vi "AUTO SIMPLE.vi"(8 "error in (no error)":errorcluster, 10 "auto command list":T1={"SHOOT\nFIRST"=FALSE, "wait to\nSHOOT (ms)"=1500, "run\nINTAKE"=FALSE, "DRIVE BRNG (deg)"=0.0, "DRIVE OUT\nVBus"=0.65, "TIME to\nDRIVE OUT (ms)"=1750, "pause after\ndrive out (ms)"=500, "SHOOT\nAGAIN"=FALSE, "DRIVE IN\nVBus"=0.0, "TIME to\nDRIVE IN (ms)"=0} {"DRIVE IN\nVBus" format="%#_13g"; "DRIVE OUT\nVBus" format="%#_13g"}) -> (0 "error out":errorcluster)   [LabVIEW 2023]
uses:
  ctrl defs/ctrl AUTO SIMPLE STEP.ctl
  ctrl defs/ctrl AUTO STEPS.ctl
  ctrl defs/ctrl FRONT FACE selector.ctl
  Global odometry.vi
  Global stack names.vi
  <vilib>/Rock Robotics/Network Tables/NT Write Boolean.vi
  <vilib>/Utility/semaphor.llb/Obtain Semaphore Reference.vi
  <vilib>/Rock Robotics/WPI/ThirdParty/JAS_Junk/TrajLib/Timer_Reset.vi
  <vilib>/Rock Robotics/WPI/ThirdParty/JAS_Junk/TrajLib/Trajectory_Library.lvlib
panel:
  out "pause after\ndrive out (ms)":u32
  out "TIME to\nDRIVE IN (ms)":u32
  out "DRIVE IN\nVBus":dbl
  out "DRIVE BRNG (deg)":u32
  out "wait to\nSHOOT (ms)":u32
  out "SHOOT\nAGAIN":bool
  out "TIME to\nDRIVE OUT (ms)":u32
  out "DRIVE OUT\nVBus":dbl
  out "run\nINTAKE":bool
  out "SHOOT\nFIRST":bool
  in  "EXIT LOOP":bool
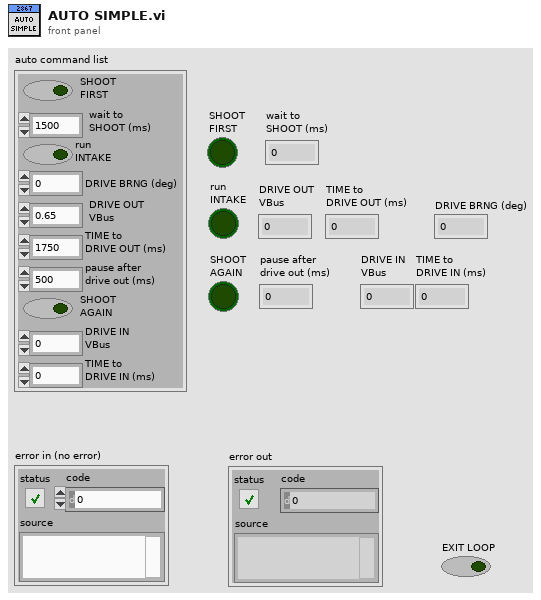
[diagram p1: front panel]
types:
  T1 = typedef "ctrl AUTO SIMPLE STEP.ctl" = cluster{"SHOOT\nFIRST":bool, "wait to\nSHOOT (ms)":u32, "run\nINTAKE":bool, "DRIVE BRNG (deg)":dbl, "DRIVE OUT\nVBus":dbl, "TIME to\nDRIVE OUT (ms)":u32, "pause after\ndrive out (ms)":u32, "SHOOT\nAGAIN":bool, "DRIVE IN\nVBus":dbl, "TIME to\nDRIVE IN (ms)":u32}
  T2 = typedef "ctrl FRONT FACE selector.ctl" = enum16{"intake side", "shooter side"}
  T3 = typedef "ctrl AUTO STEPS.ctl" = enum16{"SHOOT", "INTAKE", "ROLL OUT", "DRIVE UP", "SHOOT AGAIN", "END", "PAUSE to SHOOT", "END DRIVE"}
  T4 = typedef "ctrl stack - INTAKE SHOOTER.ctl" = cluster{"INTAKE STATE":string, "RUN INTAKE?":string, "RUN REVERSE?":string, "NOTE LOADED?":string, "SHOOTER STATE":string, "SHOOTER FIRE?":string, "SHOOT AMP?":string, "EXTEND FLAP?":string, "LOOKING for NOTE":string, "OVERIDE NOTE CHECK":string}
  T5 = typedef "Trajectory_Library.lvlib/TIMER.ctl" = cluster{"StartTime":dbl, "Accumulated TIme":dbl, "Running":bool, "semaphore":T6}
  T6 = typedef "Semaphore RefNum" = refnum<k1>
  T7 = typedef "ctrl driver input.ctl" = cluster{"Jx":dbl, "Jy":dbl, "Jr ":dbl, "R":dbl, "theta (deg)":dbl, "theta (rad)":dbl, "PARK":bool}
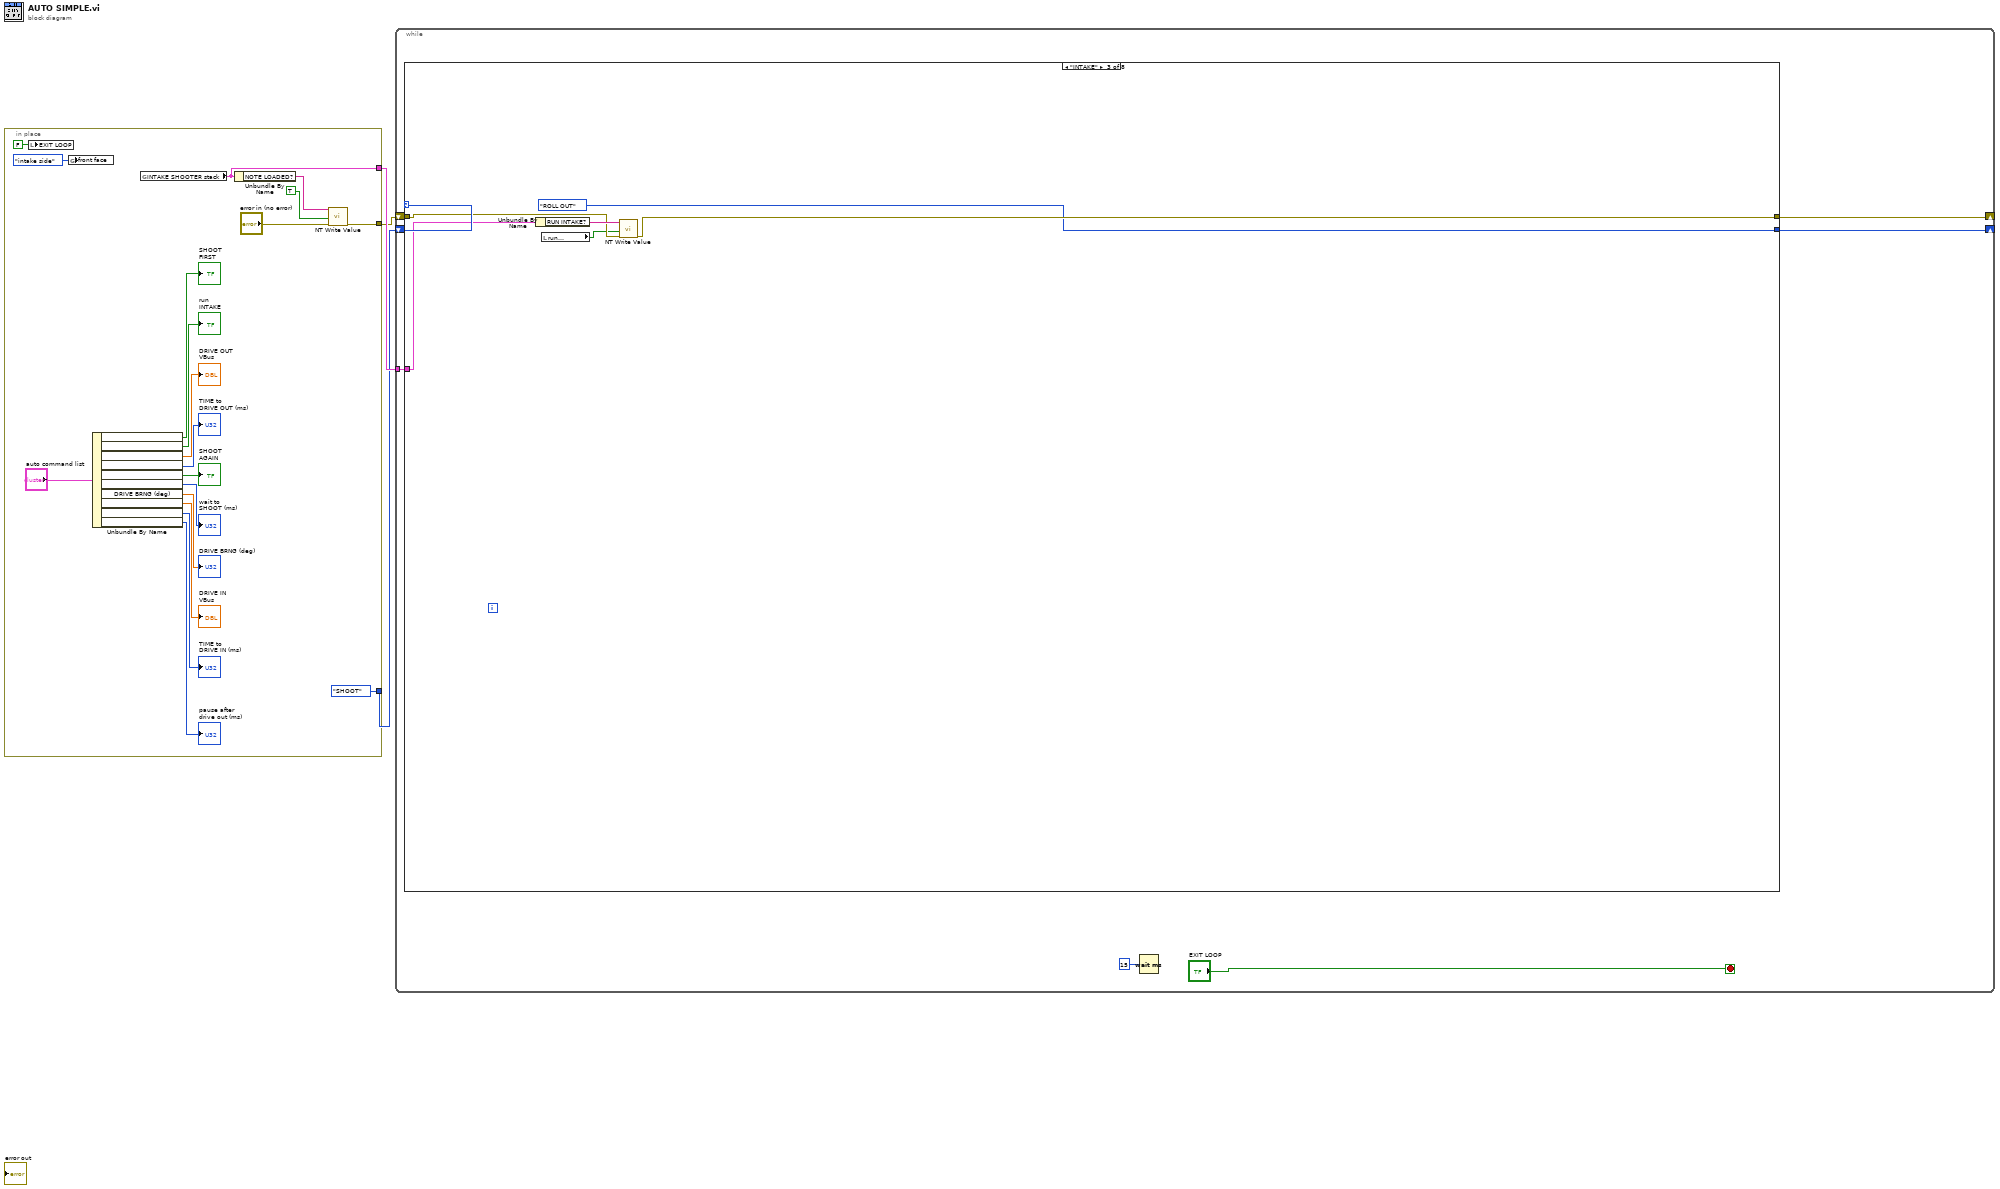
[diagram p0: block diagram]
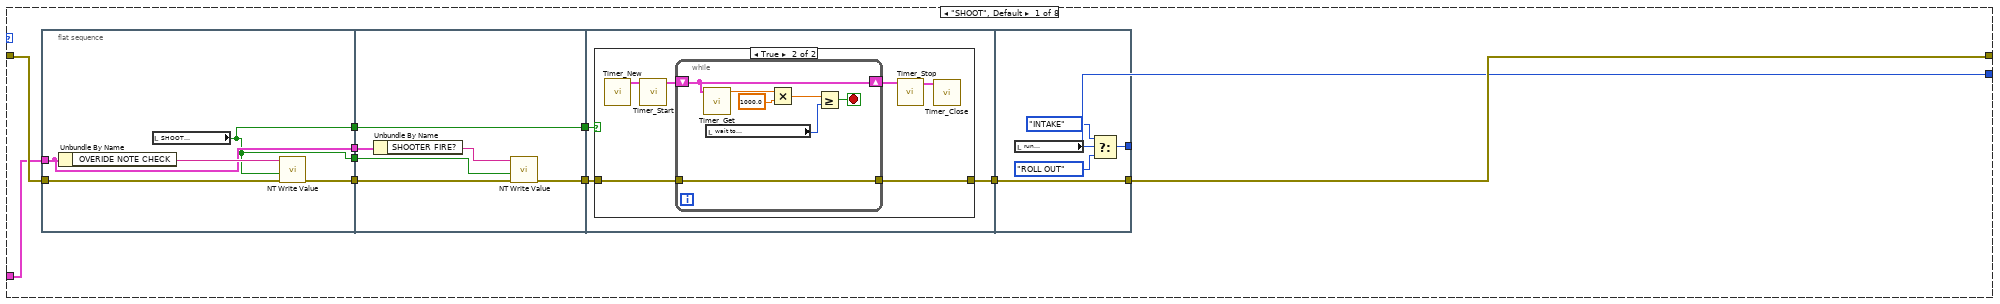
[diagram p2: hidden frame]
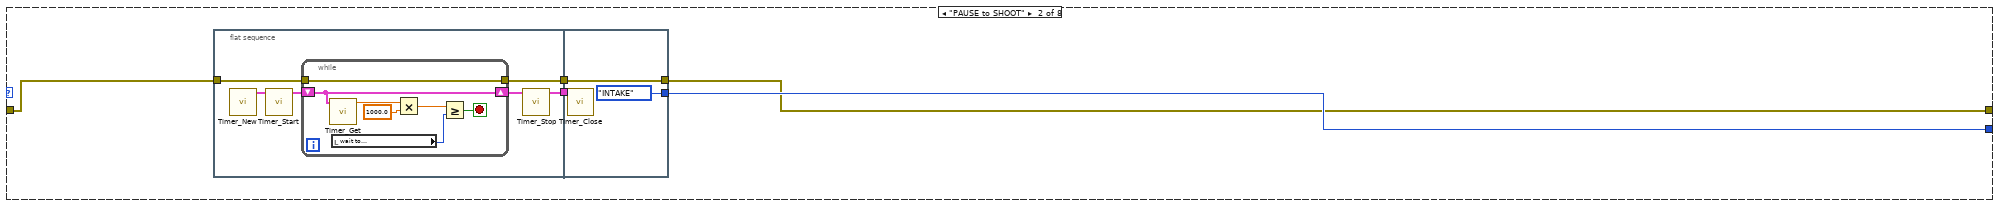
[diagram p4: hidden frame]
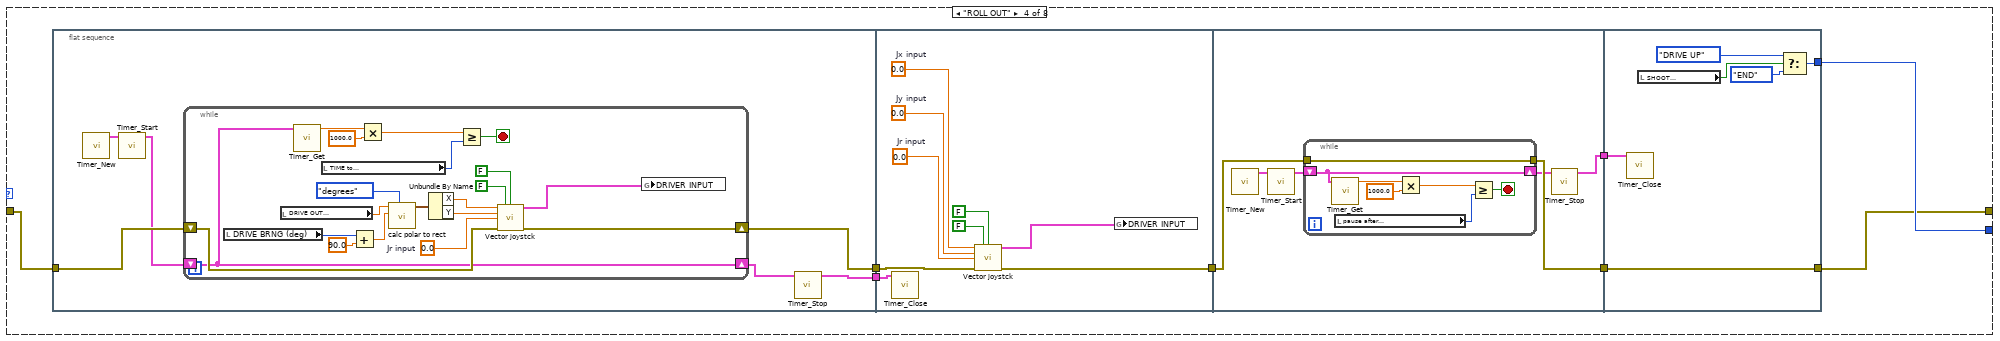
[diagram p5: hidden frame]
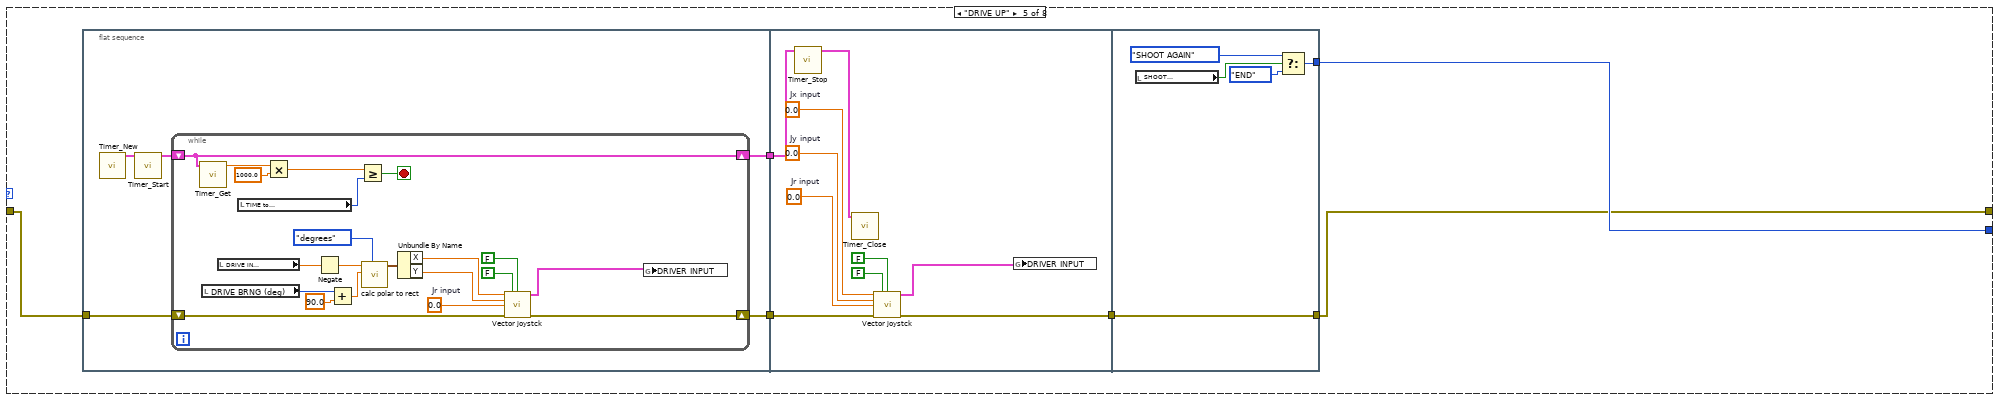
[diagram p6: hidden frame]
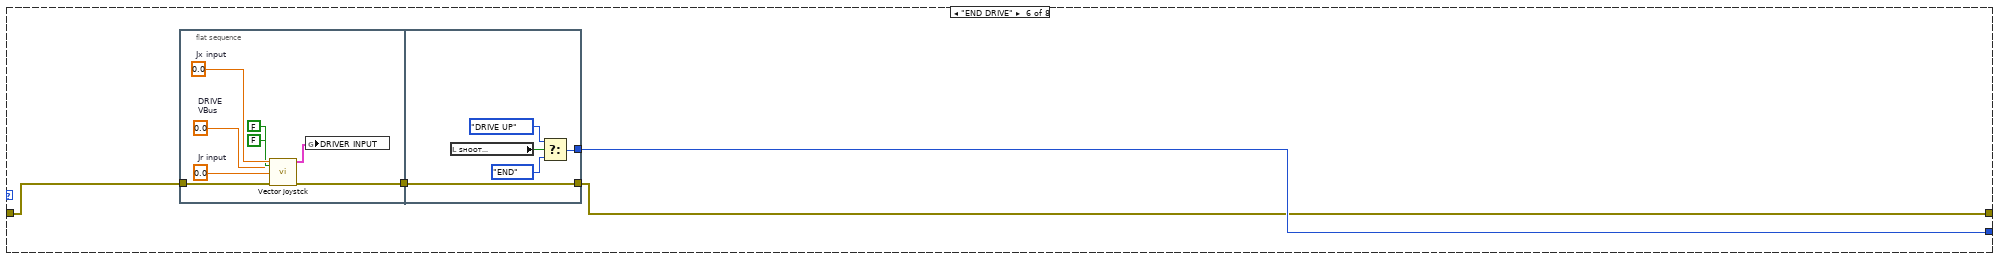
[diagram p7: hidden frame]
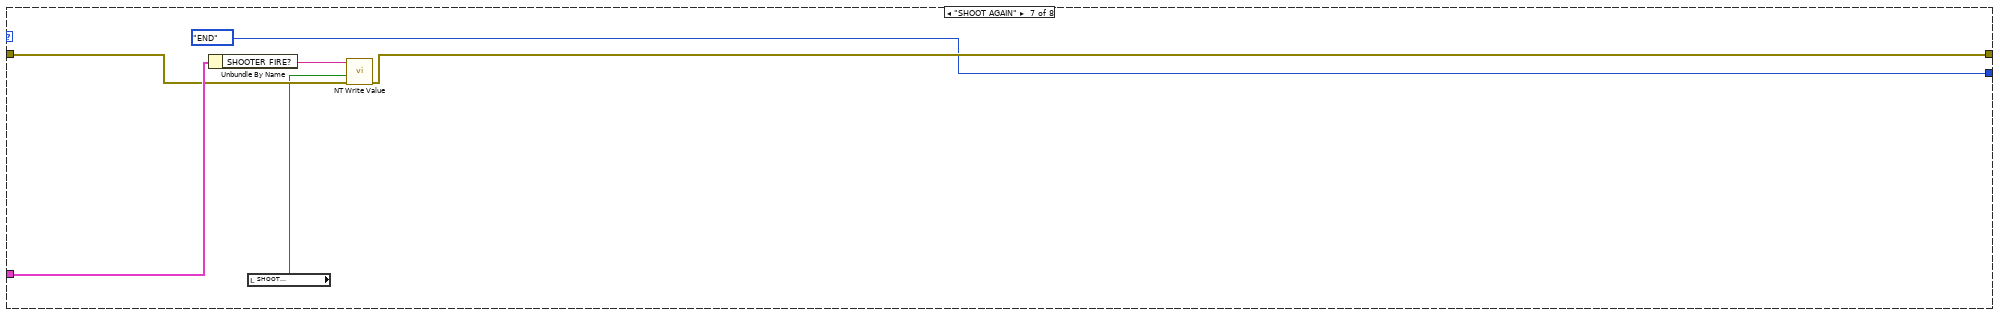
[diagram p8: hidden frame]
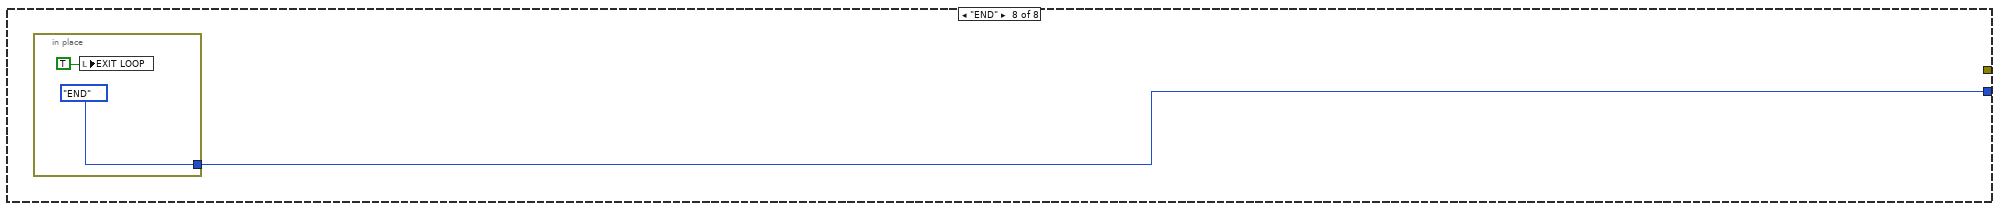
[diagram p9: hidden frame]
diagram:
  n1 = in-place {
    in-place-border: [w14] -> w3
    in-place-border: [w9] -> w2
    in-place-border: [ctrl_AUTO_STEPS."SHOOT"] -> w1
    n2 = local write "EXIT LOOP"(FALSE ("EXIT LOOP")) -> ()
    n3 = global write "Global odometry.vi" "front face"(ctrl_FRONT_FACE_selector."intake side" ("front face")) -> ()
    n4 = Unbundle By Name("auto command list") -> ("SHOOT\nFIRST"=→"SHOOT\nFIRST":bool, "run\nINTAKE"=→"run\nINTAKE":bool, "DRIVE OUT\nVBus"=→"DRIVE OUT\nVBus":dbl, "TIME to\nDRIVE OUT (ms)"=→"TIME to\nDRIVE OUT (ms)":u32, "SHOOT\nAGAIN"=→"SHOOT\nAGAIN":bool, "wait to\nSHOOT (ms)"=→"wait to\nSHOOT (ms)":u32, "DRIVE BRNG (deg)"=→"DRIVE BRNG (deg)":dbl, "DRIVE IN\nVBus"=→"DRIVE IN\nVBus":dbl, "TIME to\nDRIVE IN (ms)"=→"TIME to\nDRIVE IN (ms)":u32, "pause after\ndrive out (ms)"=→"pause after\ndrive out (ms)":u32)
    n5 = global read "Global stack names.vi" "INTAKE SHOOTER stack"() -> (w14:T4)
    n6 = Unbundle By Name(w14) -> ("NOTE LOADED?"=w13:string)
    n7 = call-poly <vilib>:"NT Write Value.vi"("error in"="error in (no error)", "value"=TRUE, "name"=w13) -> ("error out"=w9:errorcluster)  [unwired: 8 in]
  }
  n8 = while {
    shift-right: [w27] -> _
    shift-left: w2 -> [w29]
    tunnel: w3 -> [w28]
    shift-right: [w25] -> _
    shift-left: w1 -> [w26]
    stop <- "EXIT LOOP" stop-if-true
    n9 = case shown="\"INTAKE\"" w26 {
      tunnel: w28 -> [w37 _ w98 _ _ _ w231 _]
      tunnel: [w40 w74 w96 w105 w165 w210 w229 _] -> w27
      tunnel: w29 -> [w39 w76 w97 w106 w166 w211 w228 _]
      tunnel: [w38 w77 ctrl_AUTO_STEPS."ROLL OUT" w107 w167 w212 ctrl_AUTO_STEPS."END" w232] -> w25
      frame "SHOOT", Default {
        n10 = flat-sequence {
          tunnel: w39 -> [w45]
          tunnel: w37 -> [w42]
          tunnel: [w43] -> w36
          tunnel: [w41] -> w35
          tunnel: [w42] -> w34
          tunnel: [w41] -> w31
          tunnel: w36 -> [w50]
          tunnel: w35 -> [w49]
          tunnel: w34 -> [w47]
          tunnel: [w48] -> w33
          tunnel: w31 -> [w46]
          tunnel: [w46] -> w30
          tunnel: w33 -> [w54]
          tunnel: [w53] -> w32
          tunnel: w30 -> [w52]
          tunnel: [w69] -> w38
          tunnel: [w72] -> w40
          tunnel: w32 -> [w72]
          frame #0 {
            n11 = Unbundle By Name(w42) -> ("OVERIDE NOTE CHECK"=w44:string)
            n12 = local read "SHOOT\nFIRST"() -> (w41:bool)
            n13 = call-poly <vilib>:"NT Write Value.vi"("error in"=w45, "value"=w41, "name"=w44) -> ("error out"=w43:errorcluster)  [unwired: 8 in]
          }
          frame #1 {
            n14 = Unbundle By Name(w47) -> ("SHOOTER FIRE?"=w51:string)
            n15 = call-poly <vilib>:"NT Write Value.vi"("error in"=w50, "value"=w49, "name"=w51) -> ("error out"=w48:errorcluster)  [unwired: 8 in]
          }
          frame #2 {
            n16 = case shown="True" w52 {
              tunnel: w54 -> [_ w57]
              tunnel: [_ w56] -> w53
              frame False {
              }
              frame True {
                n17 = call <vilib>:"Timer_New.vi"() -> ("TIMER"=w58:T5)  [unwired: 11 in]
                n18 = call <vilib>:"Timer_Start.vi"("in Timer"=w58) -> ("out Timer"=w59:T5)  [unwired: 10 in]
                n19 = while {
                  shift-right: [w67] -> w60
                  shift-left: w59 -> [w67]
                  tunnel: w57 -> [w61]
                  tunnel: [w61] -> w56
                  stop <- w66 stop-if-true
                  n20 = call <vilib>:"Timer_Get.vi"("TIMER"=w67) -> ("CurrentTImer"=w65:dbl)  [unwired: 10 in]
                  n21 = local read "wait to\nSHOOT (ms)"() -> (w64:u32)
                  n22 = Multiply(x=w65, y=1000.0) -> (x*y=w63:dbl)
                  n23 = Greater Or Equal?(x=w63, y=w64) -> (x >= y?=w66:bool)
                }
                n24 = call <vilib>:"Timer_Stop.vi"("in Timer"=w60) -> ("out Timer"=w55:T5)  [unwired: 10 in]
                n25 = call <vilib>:"Timer_Close.vi"("TIMER"=w55) -> ()  [unwired: 11 in]
              }
            }
          }
          frame #3 {
            n26 = local read "run\nINTAKE"() -> (w68:bool)
            n27 = Select(t=ctrl_AUTO_STEPS."INTAKE", s=w68, f=ctrl_AUTO_STEPS."ROLL OUT") -> (s? t:f=w69:T3)
          }
        }
      }
      frame "PAUSE to SHOOT" {
        n28 = flat-sequence {
          tunnel: w76 -> [w80]
          tunnel: [w79] -> w75
          tunnel: [w78] -> w73
          tunnel: [ctrl_AUTO_STEPS."INTAKE"] -> w77
          tunnel: w75 -> [w92]
          tunnel: [w92] -> w74
          tunnel: w73 -> [w91]
          frame #0 {
            n29 = call <vilib>:"Timer_New.vi"() -> ("TIMER"=w81:T5)  [unwired: 11 in]
            n30 = call <vilib>:"Timer_Start.vi"("in Timer"=w81) -> ("out Timer"=w82:T5)  [unwired: 10 in]
            n31 = while {
              shift-right: [w86] -> w83
              shift-left: w82 -> [w86]
              tunnel: w80 -> [w84]
              tunnel: [w84] -> w79
              stop <- w85 stop-if-true
              n32 = call <vilib>:"Timer_Get.vi"("TIMER"=w86) -> ("CurrentTImer"=w90:dbl)  [unwired: 10 in]
              n33 = local read "wait to\nSHOOT (ms)"() -> (w89:u32)
              n34 = Multiply(x=w90, y=1000.0) -> (x*y=w88:dbl)
              n35 = Greater Or Equal?(x=w88, y=w89) -> (x >= y?=w85:bool)
            }
            n36 = call <vilib>:"Timer_Stop.vi"("in Timer"=w83) -> ("out Timer"=w78:T5)  [unwired: 10 in]
          }
          frame #1 {
            n37 = call <vilib>:"Timer_Close.vi"("TIMER"=w91) -> ()  [unwired: 11 in]
          }
        }
      }
      frame "INTAKE" {
        n38 = Unbundle By Name(w98) -> ("RUN INTAKE?"=w99:string)
        n39 = local read "run\nINTAKE"() -> (w94:bool)
        n40 = call-poly <vilib>:"NT Write Value.vi"("error in"=w97, "value"=w94, "name"=w99) -> ("error out"=w96:errorcluster)  [unwired: 8 in]
      }
      frame "ROLL OUT" {
        n41 = flat-sequence {
          tunnel: w106 -> [w113]
          tunnel: [w112] -> w102
          tunnel: [w108] -> w101
          tunnel: w102 -> [w137]
          tunnel: [w136] -> w104
          tunnel: w101 -> [w135]
          tunnel: w104 -> [w147]
          tunnel: [w146] -> w103
          tunnel: [w143] -> w100
          tunnel: [w161] -> w107
          tunnel: w103 -> [w158]
          tunnel: [w158] -> w105
          tunnel: w100 -> [w156]
          frame #0 {
            n42 = call <vilib>:"Timer_New.vi"() -> ("TIMER"=w111:T5)  [unwired: 11 in]
            n43 = call <vilib>:"Timer_Start.vi"("in Timer"=w111) -> ("out Timer"=w110:T5)  [unwired: 10 in]
            n44 = while {
              shift-right: [w130] -> w112
              shift-left: w113 -> [w131]
              shift-right: [w117] -> w109
              shift-left: w110 -> [w117]
              stop <- w115 stop-if-true
              w129 = 0.0  # Jr input
              n45 = local read "DRIVE BRNG (deg)"() -> (w125:u32)
              n46 = local read "DRIVE OUT\nVBus"() -> (w127:dbl)
              n47 = call <vilib>:"Timer_Get.vi"("TIMER"=w117) -> ("CurrentTImer"=w119:dbl)  [unwired: 10 in]
              n48 = local read "TIME to\nDRIVE OUT (ms)"() -> (w116:u32)
              n49 = Add(x=w125, y=90.0) -> (x+y=w126:dbl)
              n50 = Multiply(x=w119, y=1000.0) -> (x*y=w120:dbl)
              n51 = call "calc polar to rect.vi"("units"=enum16{"degrees", "radians"}."degrees", "angle"=w126, "mag"=w127) -> ("XY"=w128:cluster{"X":dbl, "Y":dbl})  [unwired: 8 in]
              n52 = Unbundle By Name(w128) -> ("X"=w122:dbl, "Y"=w121:dbl)
              n53 = Greater Or Equal?(x=w120, y=w116) -> (x >= y?=w115:bool)
              n54 = call "Vector joystck.vi"("Jx input"=w122, "apply\nFILTER"=FALSE ("apply\nFILTER"), "Reset\nFILTER"=FALSE ("Reset\nFILTER"), "Jy input"=w121, "Jr input"=w129, "error in (no error)"=w131) -> ("output cluster"=w114:T7, "error out"=w130:errorcluster)  [unwired: 8 in]
              n55 = global write "Global odometry.vi" "DRIVER INPUT"(w114) -> ()
            }
            n56 = call <vilib>:"Timer_Stop.vi"("in Timer"=w109) -> ("out Timer"=w108:T5)  [unwired: 10 in]
          }
          frame #1 {
            w138 = 0.0  # Jy input
            w139 = 0.0  # Jr input
            w142 = 0.0  # Jx input
            n57 = call <vilib>:"Timer_Close.vi"("TIMER"=w135) -> ()  [unwired: 11 in]
            n58 = call "Vector joystck.vi"("Jx input"=w142, "apply\nFILTER"=FALSE ("apply\nFILTER"), "Reset\nFILTER"=FALSE ("Reset\nFILTER"), "Jy input"=w138, "Jr input"=w139, "error in (no error)"=w137) -> ("output cluster"=w134:T7, "error out"=w136:errorcluster)  [unwired: 8 in]
            n59 = global write "Global odometry.vi" "DRIVER INPUT"(w134) -> ()
          }
          frame #2 {
            n60 = call <vilib>:"Timer_New.vi"() -> ("TIMER"=w148:T5)  [unwired: 11 in]
            n61 = call <vilib>:"Timer_Start.vi"("in Timer"=w148) -> ("out Timer"=w145:T5)  [unwired: 10 in]
            n62 = while {
              tunnel: w147 -> [w153]
              tunnel: [w153] -> w146
              shift-right: [w152] -> w144
              shift-left: w145 -> [w152]
              stop <- w155 stop-if-true
              n63 = call <vilib>:"Timer_Get.vi"("TIMER"=w152) -> ("CurrentTImer"=w151:dbl)  [unwired: 10 in]
              n64 = local read "pause after\ndrive out (ms)"() -> (w154:u32)
              n65 = Multiply(x=w151, y=1000.0) -> (x*y=w150:dbl)
              n66 = Greater Or Equal?(x=w150, y=w154) -> (x >= y?=w155:bool)
            }
            n67 = call <vilib>:"Timer_Stop.vi"("in Timer"=w144) -> ("out Timer"=w143:T5)  [unwired: 10 in]
          }
          frame #3 {
            n68 = call <vilib>:"Timer_Close.vi"("TIMER"=w156) -> ()  [unwired: 11 in]
            n69 = local read "SHOOT\nAGAIN"() -> (w157:bool)
            n70 = Select(t=ctrl_AUTO_STEPS."DRIVE UP", s=w157, f=ctrl_AUTO_STEPS."END") -> (s? t:f=w161:T3)
          }
        }
      }
      frame "DRIVE UP" {
        n71 = flat-sequence {
          tunnel: w166 -> [w172]
          tunnel: [w171] -> w163
          tunnel: [w168] -> w162
          tunnel: w163 -> [w198]
          tunnel: [w197] -> w164
          tunnel: w162 -> [w195]
          tunnel: [w208] -> w167
          tunnel: w164 -> [w205]
          tunnel: [w205] -> w165
          frame #0 {
            n72 = call <vilib>:"Timer_New.vi"() -> ("TIMER"=w170:T5)  [unwired: 11 in]
            n73 = call <vilib>:"Timer_Start.vi"("in Timer"=w170) -> ("out Timer"=w169:T5)  [unwired: 10 in]
            n74 = while {
              shift-right: [w189] -> w171
              shift-left: w172 -> [w190]
              shift-right: [w179] -> w168
              shift-left: w169 -> [w179]
              stop <- w178 stop-if-true
              w191 = 0.0  # Jr input
              n75 = call <vilib>:"Timer_Get.vi"("TIMER"=w179) -> ("CurrentTImer"=w177:dbl)  [unwired: 10 in]
              n76 = local read "DRIVE BRNG (deg)"() -> (w188:u32)
              n77 = local read "DRIVE IN\nVBus"() -> (w186:dbl)
              n78 = local read "TIME to\nDRIVE IN (ms)"() -> (w174:u32)
              n79 = Multiply(x=w177, y=1000.0) -> (x*y=w176:dbl)
              n80 = Negate(x=w186) -> (-x=w187:dbl)
              n81 = Add(x=w188, y=90.0) -> (x+y=w185:dbl)
              n82 = Greater Or Equal?(x=w176, y=w174) -> (x >= y?=w178:bool)
              n83 = call "calc polar to rect.vi"("units"=enum16{"degrees", "radians"}."degrees", "angle"=w185, "mag"=w187) -> ("XY"=w184:cluster{"X":dbl, "Y":dbl})  [unwired: 8 in]
              n84 = Unbundle By Name(w184) -> ("X"=w181:dbl, "Y"=w180:dbl)
              n85 = call "Vector joystck.vi"("Jx input"=w181, "apply\nFILTER"=FALSE ("apply\nFILTER"), "Reset\nFILTER"=FALSE ("Reset\nFILTER"), "Jy input"=w180, "Jr input"=w191, "error in (no error)"=w190) -> ("output cluster"=w173:T7, "error out"=w189:errorcluster)  [unwired: 8 in]
              n86 = global write "Global odometry.vi" "DRIVER INPUT"(w173) -> ()
            }
          }
          frame #1 {
            w199 = 0.0  # Jy input
            w200 = 0.0  # Jr input
            w203 = 0.0  # Jx input
            n87 = call <vilib>:"Timer_Stop.vi"("in Timer"=w195) -> ("out Timer"=w196:T5)  [unwired: 10 in]
            n88 = call <vilib>:"Timer_Close.vi"("TIMER"=w196) -> ()  [unwired: 11 in]
            n89 = call "Vector joystck.vi"("Jx input"=w203, "apply\nFILTER"=FALSE ("apply\nFILTER"), "Reset\nFILTER"=FALSE ("Reset\nFILTER"), "Jy input"=w199, "Jr input"=w200, "error in (no error)"=w198) -> ("output cluster"=w194:T7, "error out"=w197:errorcluster)  [unwired: 8 in]
            n90 = global write "Global odometry.vi" "DRIVER INPUT"(w194) -> ()
          }
          frame #2 {
            n91 = local read "SHOOT\nAGAIN"() -> (w204:bool)
            n92 = Select(t=ctrl_AUTO_STEPS."SHOOT AGAIN", s=w204, f=ctrl_AUTO_STEPS."END") -> (s? t:f=w208:T3)
          }
        }
      }
      frame "END DRIVE" {
        n93 = flat-sequence {
          tunnel: w211 -> [w215]
          tunnel: [w214] -> w209
          tunnel: [w225] -> w212
          tunnel: w209 -> [w222]
          tunnel: [w222] -> w210
          frame #0 {
            w217 = 0.0  # DRIVE VBus
            w216 = 0.0  # Jr input
            w220 = 0.0  # Jx input
            n94 = call "Vector joystck.vi"("Jx input"=w220, "apply\nFILTER"=FALSE ("apply\nFILTER"), "Reset\nFILTER"=FALSE ("Reset\nFILTER"), "Jy input"=w217, "Jr input"=w216, "error in (no error)"=w215) -> ("output cluster"=w213:T7, "error out"=w214:errorcluster)  [unwired: 8 in]
            n95 = global write "Global odometry.vi" "DRIVER INPUT"(w213) -> ()
          }
          frame #1 {
            n96 = local read "SHOOT\nAGAIN"() -> (w221:bool)
            n97 = Select(t=ctrl_AUTO_STEPS."DRIVE UP", s=w221, f=ctrl_AUTO_STEPS."END") -> (s? t:f=w225:T3)
          }
        }
      }
      frame "SHOOT AGAIN" {
        n98 = Unbundle By Name(w231) -> ("SHOOTER FIRE?"=w230:string)
        n99 = local read "SHOOT\nAGAIN"() -> (w226:bool)
        n100 = call-poly <vilib>:"NT Write Value.vi"("error in"=w228, "value"=w226, "name"=w230) -> ("error out"=w229:errorcluster)  [unwired: 8 in]
      }
      frame "END" {
        n101 = in-place {
          in-place-border: [ctrl_AUTO_STEPS."END"] -> w232
          n102 = local write "EXIT LOOP"(TRUE ("EXIT LOOP")) -> ()
        }
      }
    }
    n103 = Wait (ms)(milliseconds to wait=u32 15) -> ()  [unwired: 1 out]
  }
